vi "Lock Report.vi"(2 "error in (no error)":errorcluster, 3 "password":string, 4 "Report Ref In":T1) -> (0 "error out":errorcluster, 1 "Report Ref Out":T1)   [LabVIEW 2026, in "XCel Report Engine.lvlib"]
doc: "Protects all worksheets in the open Excel report against user modification.\n\nThe specified password is applied to every worksheet in the workbook. Calling this VI repeatedly does not create duplicate protection settings.\n\nThis protection is intended to discourage casual or unauthorized changes to generated reports. It is not a cryptographically secure mechanism and must not be treated as protection against deliberate file manipulation.\n\nUse Unlock Report.vi to remove the worksheet protection."
uses:
  XCel Report Engine.lvlib
  Controls/Report Ref.ctl
  C:/Users/weird/Desktop/XCelReportEngine/LV/DotNet/XCelReportEngine.dll
  DotNet/XCelReportEngine.dll
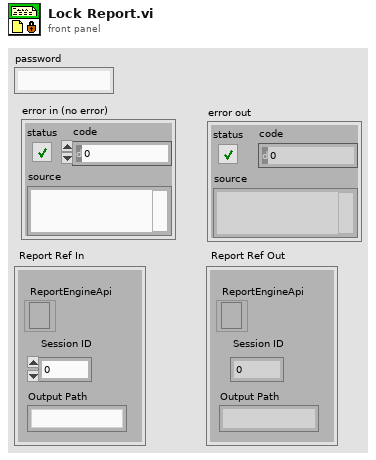
[diagram p1: front panel]
types:
  T1 = typedef "XCel Report Engine.lvlib/Report Ref.ctl" = cluster{"Session ID":i32, "Output Path":string, "ReportEngineApi":refnum<k24>}
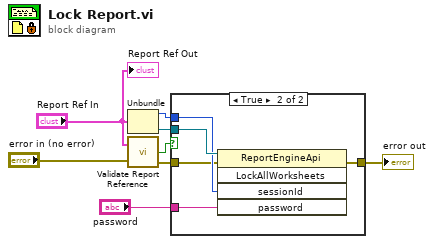
[diagram p0: block diagram]
diagram:
  n1 = Unbundle("Report Ref In") -> ("Session ID"=w5:i32, "ReportEngineApi"=w8:refnum<k24>)  [unwired: 1 out]
  n2 = call "Validate Report Reference.vi"("Report Ref In"="Report Ref In", "error in (no error)"="error in (no error)") -> ("Valid"=w1:bool, "error out"=w2:errorcluster)  [unwired: 1 out]
  n3 = case shown="True" w1 {
    tunnel: w8 -> [_ w14]
    tunnel: [w9 w13] -> w7
    tunnel: "password" -> [_ w12]
    tunnel: w5 -> [_ w11]
    tunnel: w2 -> [w9 w10]
    frame False {
    }
    frame True {
      n4 = invoke class="ReportEngineApi" method="LockAllWorksheets"(reference=w14, error in=w10, "sessionId"=w11, "password"=w12) -> (error out=w13:errorcluster)  [unwired: 1 in, 4 out]
    }
  }
  "error out" <- w7
  "Report Ref Out" <- "Report Ref In"
